vi "Insert Control Point.vi"(0 "FSM.Edge In":refnum<class "FSM.Edge.lvclass">, 7 "Even space":bool=TRUE, 9 "location":T1) -> (4 "FSM.Edge Out":refnum<class "FSM.Edge.lvclass">)   [LabVIEW 2020, in "FSM.Edge.lvclass"]
uses:
  FSM.Edge.lvclass
  <vilib>/Utility/miscctls.llb/LVPoint32TypeDef.ctl
  FSM.Edge.lvclass/FSM.Edge.ctl
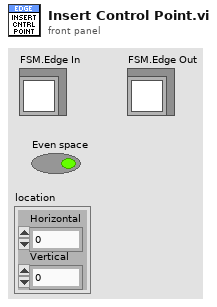
[diagram p1: front panel]
types:
  T1 = typedef "LVPoint32TypeDef.ctl" = cluster{"Horizontal":i32, "Vertical":i32}
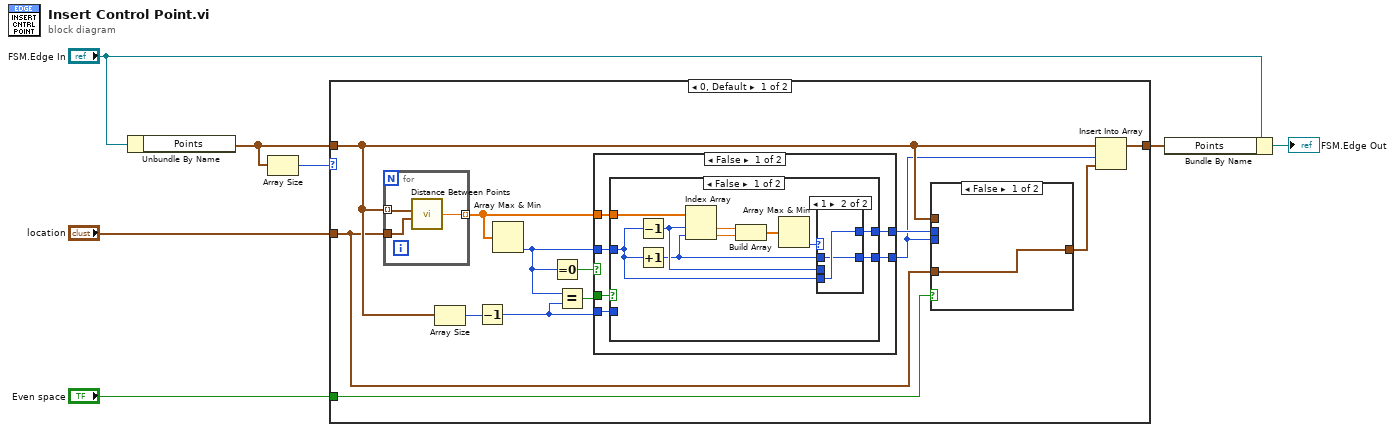
[diagram p0: block diagram]
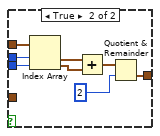
[diagram p2: hidden frame]
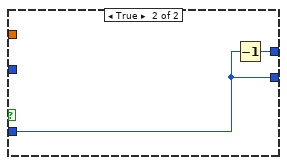
[diagram p4: hidden frame]
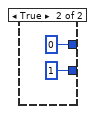
[diagram p5: hidden frame]
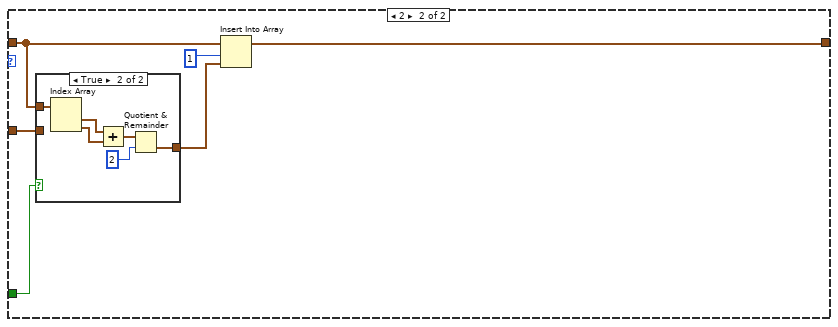
[diagram p6: hidden frame]
diagram:
  n1 = Unbundle By Name("FSM.Edge In") -> ("Points"=w3:cluster{"x":i16, "y":i16}[])
  n2 = Array Size(array=w3) -> (size(s)=w2:i32)
  n3 = case shown="0, Default" w2 {
    tunnel: "location" -> [w9 w57]
    tunnel: [w19 w61] -> w4
    tunnel: w3 -> [w16 w62]
    tunnel: "Even space" -> [w8 w58]
    frame 0, Default {
      n4 = for {
        tunnel: w16 -> [w56] mode=indexing
        tunnel: w9 -> [w55]
        tunnel: [w54] -> w12 mode=indexing
        n5 = call "Distance Between Points.vi"("B"=w55, "A"=w56) -> ("distance"=w54:dbl)  [unwired: 4 in]
      }
      n6 = Array Size(array=w16) -> (size(s)=w15:i32)
      n7 = Decrement(x=w15) -> (x-1=w13:i32)
      n8 = Array Max & Min(array=w12) -> (min index (indices)=w11:i32)  [unwired: 3 out]
      n9 = Equal To 0?(x=w11) -> (x = 0?=w20:bool)
      n10 = Equal?(x=w11, y=w13) -> (x = y?=w14:bool)
      n11 = case shown="False" w20 {
        tunnel: [w35 0] -> w17
        tunnel: [w34 1] -> w10
        tunnel: w14 -> [w33 _]
        tunnel: w13 -> [w32 _]
        tunnel: w12 -> [w31 _]
        tunnel: w11 -> [w30 _]
        frame False {
          n12 = case shown="False" w33 {
            tunnel: [w37 w51] -> w35
            tunnel: [w40 w50] -> w34
            tunnel: w32 -> [_ w50]
            tunnel: w31 -> [w45 _]
            tunnel: w30 -> [w39 _]
            frame False {
              n13 = Decrement(x=w39) -> (x-1=w38:i32)
              n14 = Increment(x=w39) -> (x+1=w36:i32)
              n15 = Index Array(array=w45, index #1=w38, index #2=w36) -> (element #1=w44:dbl, element #2=w43:dbl)
              n16 = Build Array(w44, w43) -> (w42:dbl[])
              n17 = Array Max & Min(array=w42) -> (min index (indices)=w41:i32)  [unwired: 3 out]
              n18 = case shown="1" w41 {
                tunnel: [w47 w48] -> w40
                tunnel: w39 -> [w47 w49]
                tunnel: w38 -> [w46 _]
                tunnel: [w46 w49] -> w37
                tunnel: w36 -> [_ w48]
                frame 0, Default {
                }
                frame 1 {
                }
              }
            }
            frame True {
              n19 = Decrement(x=w50) -> (x-1=w51:i32)
            }
          }
        }
        frame True {
        }
      }
      n20 = case shown="False" w8 {
        tunnel: [w21 w25] -> w18
        tunnel: w17 -> [_ w24]
        tunnel: w16 -> [_ w23]
        tunnel: w10 -> [_ w22]
        tunnel: w9 -> [w21 _]
        frame False {
        }
        frame True {
          n21 = Index Array(array=w23, index #1=w24, index #2=w22) -> (element #1=w29:cluster{"x":i16, "y":i16}, element #2=w28:cluster{"x":i16, "y":i16})
          n22 = Add(x=w29, y=w28) -> (x+y=w27:cluster{"x":i16, "y":i16})
          n23 = Quotient & Remainder(x=w27, y=2) -> (floor(x/y)=w25:cluster{"x":i32, "y":i32})  [unwired: 1 out]
        }
      }
      n24 = Insert Into Array(array=w16, index=w10, new element=w18) -> (w19:cluster{"x":i16, "y":i16}[])
    }
    frame 2 {
      n25 = case shown="True" w58 {
        tunnel: w62 -> [_ w65]
        tunnel: [w63 w64] -> w60
        tunnel: w57 -> [w63 _]
        frame False {
        }
        frame True {
          n26 = Index Array(array=w65) -> (element #1=w69:cluster{"x":i16, "y":i16}, element #2=w68:cluster{"x":i16, "y":i16})  [unwired: 2 in]
          n27 = Add(x=w69, y=w68) -> (x+y=w67:cluster{"x":i16, "y":i16})
          n28 = Quotient & Remainder(x=w67, y=2) -> (floor(x/y)=w64:cluster{"x":i32, "y":i32})  [unwired: 1 out]
        }
      }
      n29 = Insert Into Array(array=w62, index=1, new element=w60) -> (w61:cluster{"x":i16, "y":i16}[])
    }
  }
  n30 = Bundle By Name(cluster="FSM.Edge In", "Points"=w4) -> (→"FSM.Edge Out":refnum<class "FSM.Edge.lvclass">)
